vi "SetParam.vi"(8 "error in (no error)":errorcluster caption="entrée d'erreur (pas d'erreur)", 10 "fetch_kddcup99":T1={"subset"="None", "shuffle"=TRUE, "random_state"=-1, "percent10"=TRUE, "download_if_missing"=TRUE, "Returns"="Data"} {"random_state" min=-1}, 11 "Kddcup99.lvclass":refnum<class "Kddcup99.lvclass">) -> (0 "error out":errorcluster caption="sortie d'erreur", 3 "Kddcup99.lvclass":refnum<class "Kddcup99.lvclass">)   [LabVIEW 2020, in "Kddcup99.lvclass"]
doc: "Set Parameters"
uses:
  Kddcup99.lvclass
  Kddcup99.lvclass/Kddcup99.ctl
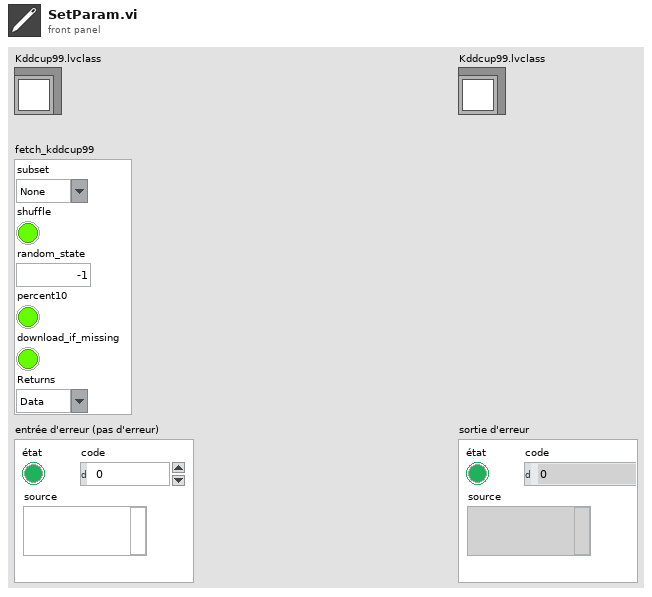
[diagram p1: front panel]
types:
  T1 = cluster{"subset":string, "shuffle":bool, "random_state":i32, "percent10":bool, "download_if_missing":bool, "Returns":string}
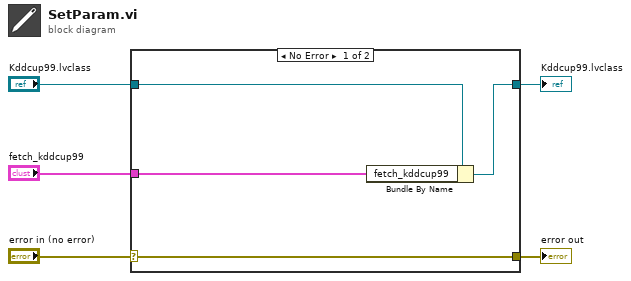
[diagram p0: block diagram]
diagram:
  n1 = case shown="No Error" "error in (no error)" {
    selector: "error in (no error)" -> [w9 w10]
    tunnel: [w9 w10] -> w4
    tunnel: [w7 w11] -> w2
    tunnel: "Kddcup99.lvclass" -> [w8 w11]
    tunnel: "fetch_kddcup99" -> [w6 _]
    frame No Error {
      n2 = Bundle By Name(cluster=w8, "fetch_kddcup99"=w6) -> (w7:refnum<class "Kddcup99.lvclass">)
    }
    frame Error {
    }
  }
  "error out" <- w4
  "Kddcup99.lvclass" <- w2
